vi "test Insert Intersection Data In Cluster Array XY Correct.vi"(8 "error in (no error)":errorcluster, 11 "TestCase in":refnum<class "Utility VIs tests.lvclass">) -> (0 "error out":errorcluster, 3 "TestCase out":refnum<class "Utility VIs tests.lvclass">)   [LabVIEW 2014, in "Utility VIs tests.lvclass"]
uses:
  Utility VIs tests.lvclass
  <vilib>/addons/_JKI Toolkits/VI Tester/TestCase.llb/TestCase.lvclass
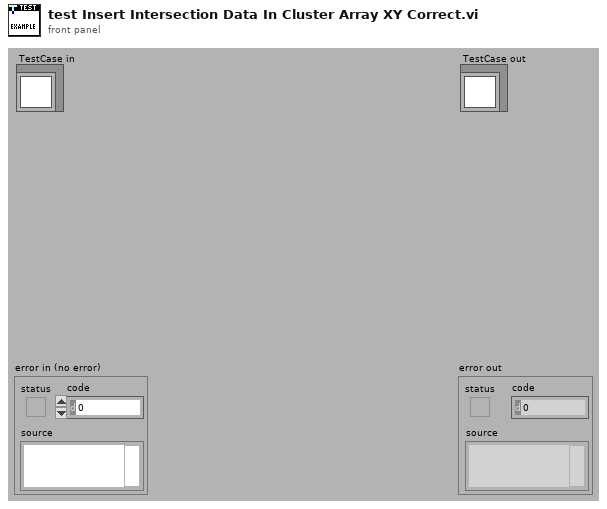
[diagram p1: front panel]
types:
  T1 = cluster{"Time [ms]":dbl, "x":dbl, "y":dbl, "Fout":bool, "Goed":bool}[]
  T2 = cluster{"Time [ms]":dbl, "x":dbl, "y":dbl, "Fout":bool, "Goed":bool}
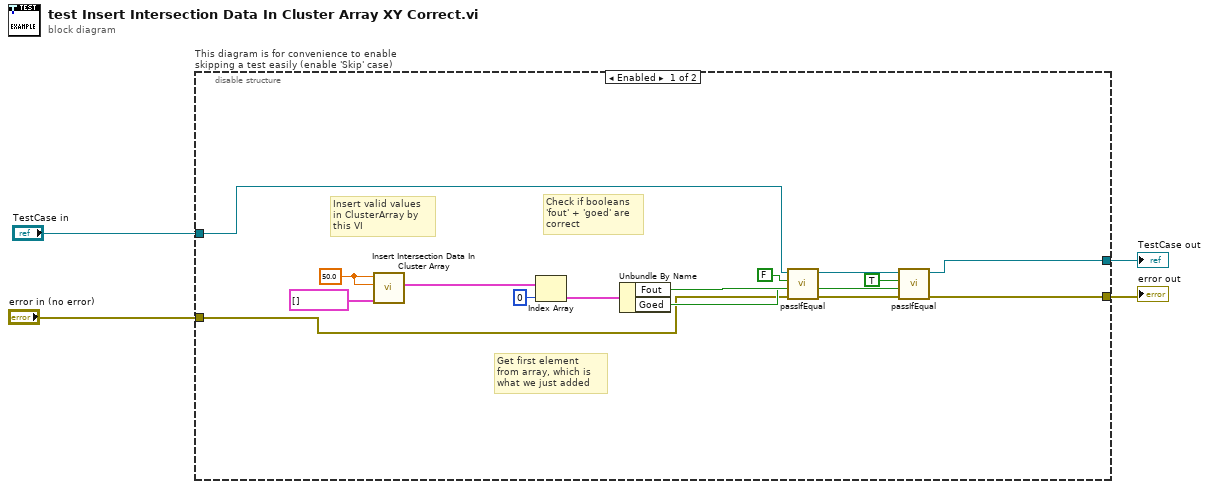
[diagram p0: block diagram]
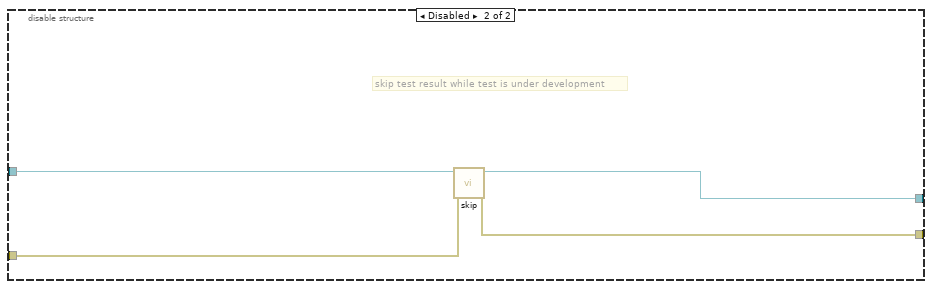
[diagram p2: hidden frame]
diagram:
  n1 = disable-structure "This diagram is for convenience to enable skipping a test easily (enable 'Skip' case)" shown="Enabled" {
    disable-tunnel: "TestCase in" -> [w10 w23]
    disable-tunnel: [w8 w21] -> w1
    disable-tunnel: [w5 w22] -> w3
    disable-tunnel: "error in (no error)" -> [w7 w20]
    frame Enabled {
      w18 = 50.0 ("X")
      # "Get first element\nfrom array, which is \nwhat we just added"
      # "Check if booleans\n'fout' + 'goed' are\ncorrect"
      # "Insert valid values\nin ClusterArray by \nthis VI"
      n2 = call "Insert Intersection Data In Cluster Array.vi"("ClusterArray"=T1 [], "Y"=w18, "X"=w18) -> ("Intersections"=w17:T1)  [unwired: 8 in]
      n3 = Index Array(array=w17, index=0) -> (element=w15:T2)
      n4 = Unbundle By Name(w15) -> ("Fout"=w14:bool, "Goed"=w13:bool)
      n5 = call-dynamic "passIfEqual.vi"("error in (no error)"=w7, "y"=w14, "x"=FALSE, "TestCase in"=w10) -> ("error out"=w6:errorcluster, "TestCase out"=w9:refnum<class "Utility VIs tests.lvclass">)  [unwired: 6 in]
      n6 = call-dynamic "passIfEqual.vi"("error in (no error)"=w6, "y"=w13, "x"=TRUE, "TestCase in"=w9) -> ("error out"=w5:errorcluster, "TestCase out"=w8:refnum<class "Utility VIs tests.lvclass">)  [unwired: 6 in]
    }
    frame Disabled {
      # "skip test result while test is under development"
      n7 = call <vilib>:"skip.vi"("error in (no error)"=w20, "TestCase in"=w23) -> ("error out"=w22:errorcluster, "TestCase out"=w21:refnum<class "Utility VIs tests.lvclass">)  [unwired: 8 in]
    }
  }
  "error out" <- w3
  "TestCase out" <- w1
